vi "Team Move v1.vi"(11 "View out":i32[](array[numeric]) caption="Updated View (-1 team, 0 empty, 1 enemy)") -> (2 "Direction":T2, 3 "Action":T1)   [LabVIEW 2020, in "Ant Mound.lvclass"]
uses:
  Ant Mound.lvclass
  Type Defs/Direction Enum.ctl
  Type Defs/Action Enum.ctl
  <vilib>/Analysis/baseanly.llb/Real Dot Product.vi
  DS Square Library/DS Square.lvlib
  <vilib>/Analysis/NI_AALBase.lvlib
  Type Defs/SB Type Defs.lvlib
panel:
  out "direction (deg)":dbl
  out "magnitude":dbl
  # "NW\nN\nNE\nE\nSE\nS\nSW\nW"
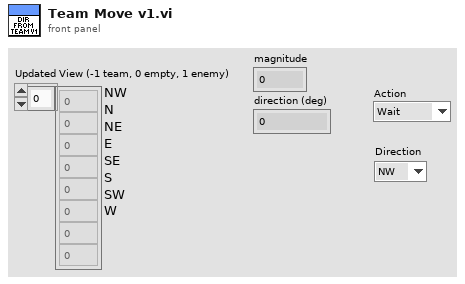
[diagram p1: front panel]
types:
  T1 = typedef "SB Type Defs.lvlib/Action Enum.ctl" = enum16{"Wait", "Move", "Attack", "Replicate"}
  T2 = typedef "SB Type Defs.lvlib/Direction Enum.ctl" = enum16{"NW", "N", "NE", "E", "SE", "S", "SW", "W"}
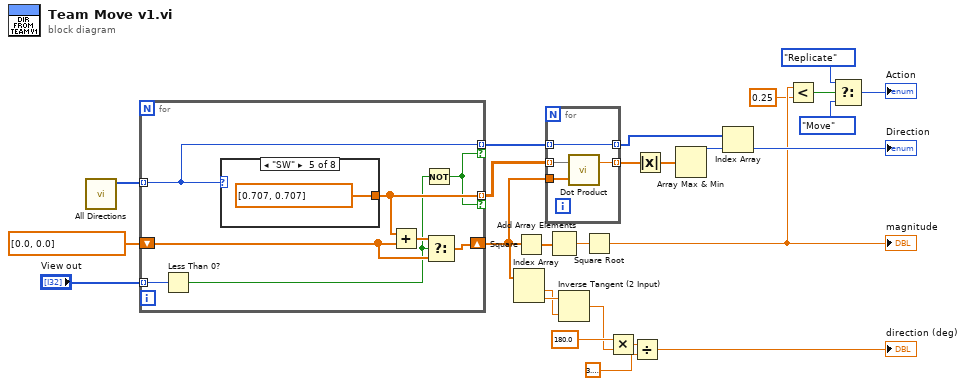
[diagram p0: block diagram]
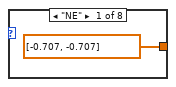
[diagram p2: hidden frame]
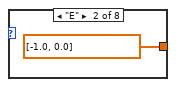
[diagram p3: hidden frame]
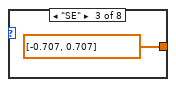
[diagram p4: hidden frame]
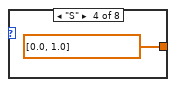
[diagram p5: hidden frame]
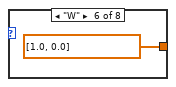
[diagram p6: hidden frame]
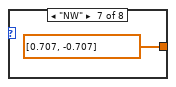
[diagram p7: hidden frame]
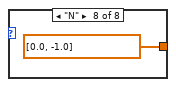
[diagram p8: hidden frame]
diagram:
  n1 = call "All Directions.vi"() -> ("All directions"=w20:T2[])  [unwired: 11 in]
  n2 = for {
    tunnel: "View out" -> [w34] mode=indexing
    shift-right: [w31] -> w13
    shift-left: dbl[] [0.0, 0.0] ("X Vector") -> [w32]
    tunnel: w20 -> [w29] mode=indexing
    tunnel: [w30] -> w14 mode=indexing if=w27
    tunnel: [w29] -> w12 mode=indexing if=w27
    n3 = Less Than 0?(x=w34) -> (x < 0?=w28:bool)
    n4 = case shown="\"SW\"" w29 {
      tunnel: [dbl[] [-0.707, -0.707] ("X Vector") dbl[] [-1.0, 0.0] ("X Vector") dbl[] [-0.707, 0.707] ("X Vector") dbl[] [0.0, 1.0] ("X Vector") dbl[] [0.707, 0.707] ("X Vector") dbl[] [1.0, 0.0] ("X Vector") dbl[] [0.707, -0.707] ("X Vector") dbl[] [0.0, -1.0] ("X Vector")] -> w30
      frame "NE" {
      }
      frame "E" {
      }
      frame "SE" {
      }
      frame "S" {
      }
      frame "SW" {
      }
      frame "W" {
      }
      frame "NW" {
      }
      frame "N" {
      }
    }
    n5 = Add(x=w30, y=w32) -> (x+y=w33:dbl[])
    n6 = Not(x=w28) -> (.not. x?=w27:bool)
    n7 = Select(t=w33, s=w28, f=w32) -> (s? t:f=w31:dbl[])
  }
  n8 = Index Array(array=w13) -> (element #1=w21:dbl, element #2=w22:dbl)  [unwired: 2 in]
  n9 = Square(x=w13) -> (x^2=w24:dbl[])
  n10 = for {
    tunnel: w14 -> [w46] mode=indexing
    tunnel: w13 -> [w45]
    tunnel: [w44] -> w2 mode=indexing
    tunnel: w12 -> [w43] mode=indexing
    tunnel: [w43] -> w11 mode=indexing
    n11 = call-poly <vilib>:"Dot Product.vi"("Y Vector"=w45, "X Vector"=w46) -> ("X * Y"=w44:dbl)  [unwired: 1 out]
  }
  n12 = Add Array Elements(numeric array=w24) -> (sum=w23:dbl)
  n13 = Inverse Tangent (2 Input)(1:w21, 2:w22) -> (0:w18:dbl)
  n14 = Square Root(x=w23) -> (sqrt(x)=w8:dbl)
  "magnitude" <- w8
  n15 = Multiply(x=180.0, y=w18) -> (x*y=w17:dbl)
  n16 = Divide(x=w17, y=3.141592653589793) -> (x/y=→"direction (deg)":dbl)
  n17 = Absolute Value(x=w2) -> (abs(x)=w1:dbl[])
  n18 = Array Max & Min(array=w1) -> (max index (indices)=w10:i32)  [unwired: 3 out]
  n19 = Index Array(array=w11, index=w10) -> (element=→"Direction":T2)
  n20 = Less?(x=w8, y=0.25) -> (x < y?=w6:bool)
  n21 = Select(t=Action_Enum."Replicate" ("Action"), s=w6, f=Action_Enum."Move" ("Action")) -> (s? t:f=→"Action":T1)
